vi "Provider_OnCommand.vi"(10 "Command ID":string, 11 "objects":T1[](array[typedef])) -> ()   [LabVIEW 2020, in "Message Maker Provider.lvlib"]
uses:
  Message Maker Provider.lvlib
  _Message Maker/Message Maker.lvlib
  <resource>/Framework/Providers/API/ItemRef.ctl
panel:
  out "error out":errorcluster
  in  "error in":errorcluster
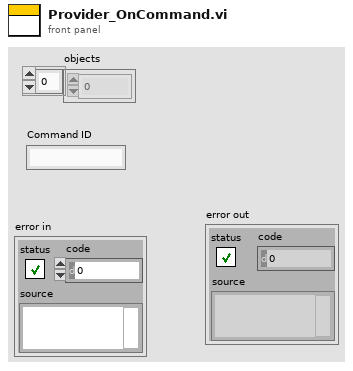
[diagram p1: front panel]
types:
  T1 = typedef "ItemRef.ctl" = u64
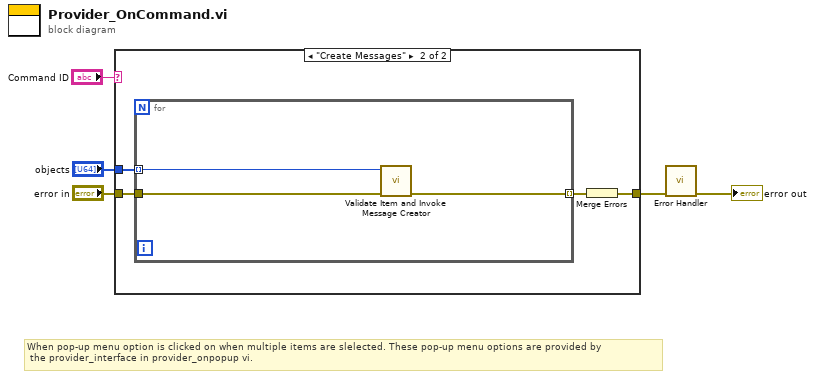
[diagram p0: block diagram]
diagram:
  # "When pop-up menu option is clicked on when multiple items are slelected. These pop-up menu options are provided by\n the provider_interface in provider_onpopup vi."
  n1 = case shown="\"Create Messages\"" "Command ID" {
    tunnel: "error in" -> [w6 w9]
    tunnel: [w6 w7] -> w1
    tunnel: "objects" -> [_ w10]
    frame Default {
    }
    frame "Create Messages" {
      n2 = for {
        tunnel: w10 -> [w13] mode=indexing
        tunnel: w9 -> [w12]
        tunnel: [w11] -> w8 mode=indexing
        n3 = call "Validate Item and Invoke Message Creator.vi"("error in (no error)"=w12, "Object"=w13) -> ("error out"=w11:errorcluster)  [unwired: 9 in]
      }
      n4 = Merge Errors(w8) -> (w7:errorcluster)
    }
  }
  n5 = call "Error Handler.vi"("error in (no error)"=w1) -> ("error out"=→"error out":errorcluster)  [unwired: 10 in]
